vi "GF_SaveAgilentData.vi"(1 "Agilent Scintillator Scope Graph":waveform(dbl)[](graph)=[{"t0"=timestamp(-9.999999999998899e-05 s since 1904-01-01), "dt"=2e-09, "Y"=array[1000000 elements]}, {"t0"=timestamp(-9.999999999998899e-05 s since 1904-01-01), "dt"=2e-09, "Y"=array[1000000 elements]}], 3 "Base Path":path) -> (0 "error out":errorcluster)   [LabVIEW 2020]
panel:
  out "Time Stamp":string
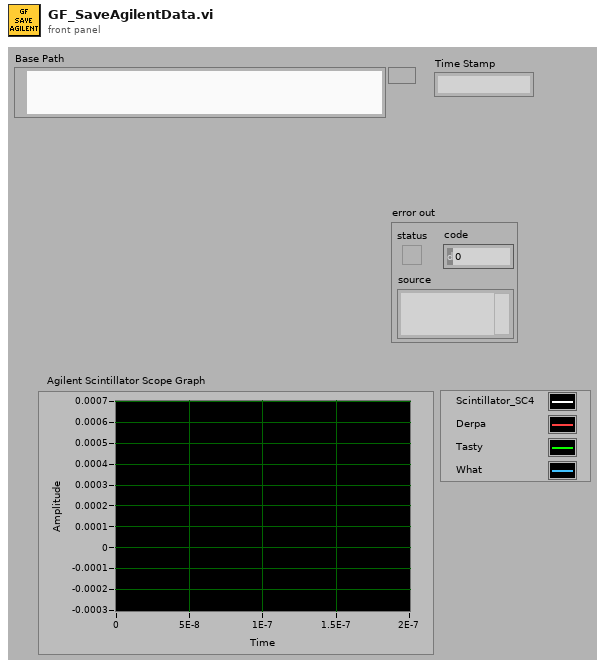
[diagram p1: front panel]
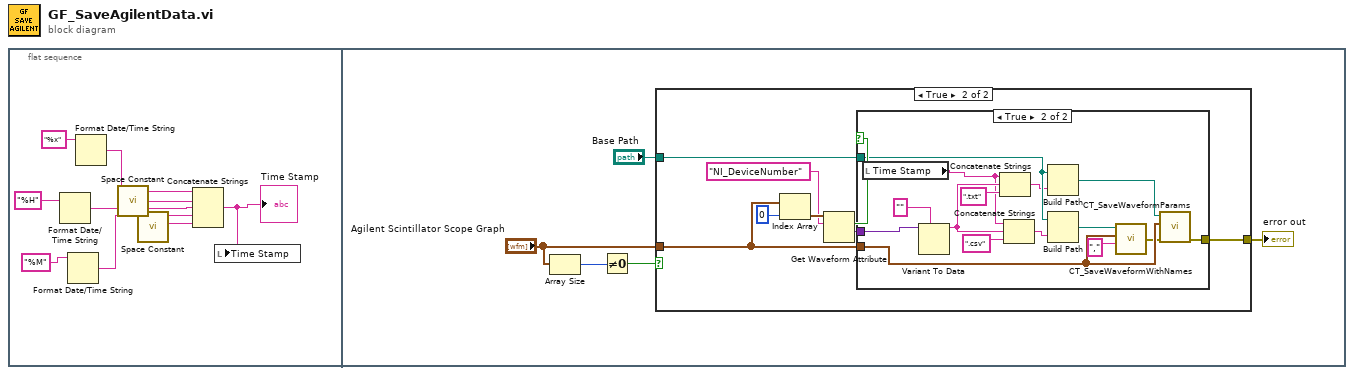
[diagram p0: block diagram]
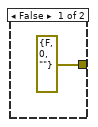
[diagram p2: hidden frame]
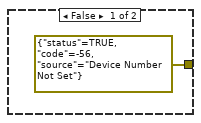
[diagram p3: hidden frame]
diagram:
  n1 = flat-sequence {
    frame #0 {
      n2 = Format Date/Time String(time format string (%c)="%H") -> (date/time string=w7:string)  [unwired: 2 in]
      n3 = Format Date/Time String(time format string (%c)="%M") -> (date/time string=w8:string)  [unwired: 2 in]
      n4 = Format Date/Time String(time format string (%c)="%x") -> (date/time string=w5:string)  [unwired: 2 in]
      n5 = call <vilib>:"Space Constant.vi"() -> ("String"=w6:string)
      n6 = call <vilib>:"Space Constant.vi"() -> ("String"=w1:string)
      n7 = Concatenate Strings(w5, w6, w7, w8, w1) -> (w9:string)
      "Time Stamp" <- w9
      n8 = local write "Time Stamp"(w9) -> ()
    }
    frame #1 {
      n9 = Array Size(array="Agilent Scintillator Scope Graph") -> (size(s)=w11:i32)
      n10 = Not Equal To 0?(x=w11) -> (x != 0?=w10:bool)
      n11 = case shown="True" w10 {
        tunnel: [errorcluster {"status"=FALSE, "code"=0, "source"=""} ("error out") w23] -> w14
        tunnel: "Base Path" -> [_ w22]
        tunnel: "Agilent Scintillator Scope Graph" -> [_ w21]
        frame False {
        }
        frame True {
          n12 = Index Array(array=w21, index=0) -> (element=w19:waveform(dbl))
          n13 = Get Waveform Attribute(6:"NI_DeviceNumber" ("name"), 7:w19) -> (1:w16:variant, 2:w17:bool)  [unwired: 2 in, 2 out]
          n14 = case shown="True" w17 {
            tunnel: [errorcluster {"status"=TRUE, "code"=-56, "source"="Device Number Not Set"} ("error out") w26] -> w23
            tunnel: w22 -> [_ w33]
            tunnel: w21 -> [_ w28]
            tunnel: w16 -> [_ w37]
            frame False {
            }
            frame True {
              n15 = local read "Time Stamp"() -> (w25:string)
              n16 = Variant To Data(type="" ("delimiter (Tab)"), Variant=w37) -> (data=w30:string)  [unwired: 1 in, 1 out]
              n17 = Concatenate Strings(w25, w30, ".txt" ("string")) -> (w31:string)
              n18 = Concatenate Strings(w25, w30, ".csv" ("string")) -> (w35:string)
              n19 = Build Path(base path=w33, name or relative path=w31) -> (appended path=w29:path)
              n20 = Build Path(base path=w33, name or relative path=w35) -> (appended path=w38:path)
              n21 = call "CT_SaveWaveformWithNames.vi"("delimiter (Tab)"=",", "waveforms"=w28, "file path (dialog if empty)"=w38) -> ("error out"=w27:errorcluster)  [unwired: 1 in]
              n22 = call "CT_SaveWaveformParams.vi"("error in (no error)"=w27, "Agilent Scintillator Scope Graph"=w28, "file path (dialog if empty)"=w29) -> ("error out"=w26:errorcluster)  [unwired: 8 in]
            }
          }
        }
      }
      "error out" <- w14
    }
  }
